vi "initialize Session Data.vi"(0 "OBJ - Session in":refnum<class "Exscalabar FPGA.lvclass">, 11 "error in":errorcluster) -> (4 "OBJ - Session out":refnum<class "Exscalabar FPGA.lvclass">, 15 "error out":errorcluster)   [LabVIEW 2014, in "Exscalabar FPGA.lvclass"]
doc: "Open an EXSCALABAR R series specific FPGA session. The system forces a wait on interrupt, so acknowledge the interrupt before moving on or the card will not respond properly. \n\nWhile the error on opening is logged, the error is further propagated so that the caller can handle the error and not just log it."
uses:
  Exscalabar FPGA.lvclass
  Exscalabar FPGA.lvclass/Exscalabar FPGA.ctl
  <vilib>/Utility/error.llb/Error Cluster From Error Code.vi
  <vilib>/rvi/errors/niLvFpgaAdjustHostInterfaceError.vi
  <vilib>/RVI Host/nirviSupport.llb/nirviErrorClusterFromErrorCode.vi
  <vilib>/rvi/interface/common/niFpgaWaitOnOcc.vi
  <vilib>/FPGAPlugInAG/PXI-7842R/niLvFpga_Open_PXI-7842R.vi
  R FPGA Ref.ctl
  <vilib>/rvi/interface/nirviMethod/nirviMethod.xnode
  FPGA Bitfiles/FPGA Server.lvbitx
  <vilib>/rvi/interface/nirviReadWriteControl/nirviReadWriteControl.xnode
  <vilib>/rvi/interface/nirviOpenFPGA/nirviOpenFPGA.xnode
  reusable/Session APIs/Session Log/System Log.lvclass
  <vilib>/rvi/errors/niLvFpgaMergeErrorWithErrorCode.vi
  <vilib>/FPGAPlugInAG/PXI-7842R/niLvFpga_ConfigureFifo_PXI-7842R.vi
  <vilib>/FPGAPlugInAG/PXI-7842R/niLvFpga_StartFifo_PXI-7842R.vi
  NiFpgaLv.dll
  <vilib>/rvi/interface/nirviMethod/StockFPGA_InlinedMethodWaitForSingleIRQ.vi
  <vilib>/FPGAPlugInAG/PXI-7842R/niLvFpga_WaitOnIrq_PXI-7842R.vi
  <vilib>/FPGAPlugInAG/PXI-7842R/niLvFpga_AcknowledgeIrq_PXI-7842R.vi
  PAS/ePAS Library.lvlib
panel:
  out "stopped":bool
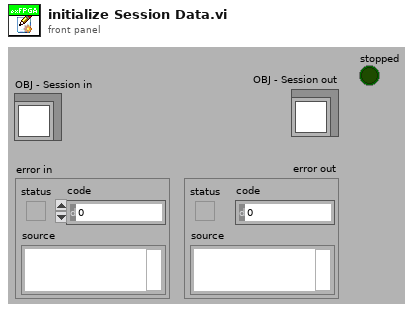
[diagram p1: front panel]
types:
  T1 = cluster{"f0":fxp<+,32,0>, "Scale":fxp<+,14,1>, "Offset":i16, "Mod":enum8{"Sine", "Square"}}
  T2 = cluster{"Ch1":bool, "Ch2":bool, "Ch3":bool, "Ch4":bool, "Ch5":bool}
  T3 = typedef "Session - Root.lvclass/Session Handle.ctl" = refnum<data-value>
  T4 = typedef "ePAS Library.lvlib/R FPGA Ref.ctl" = refnum<k20>
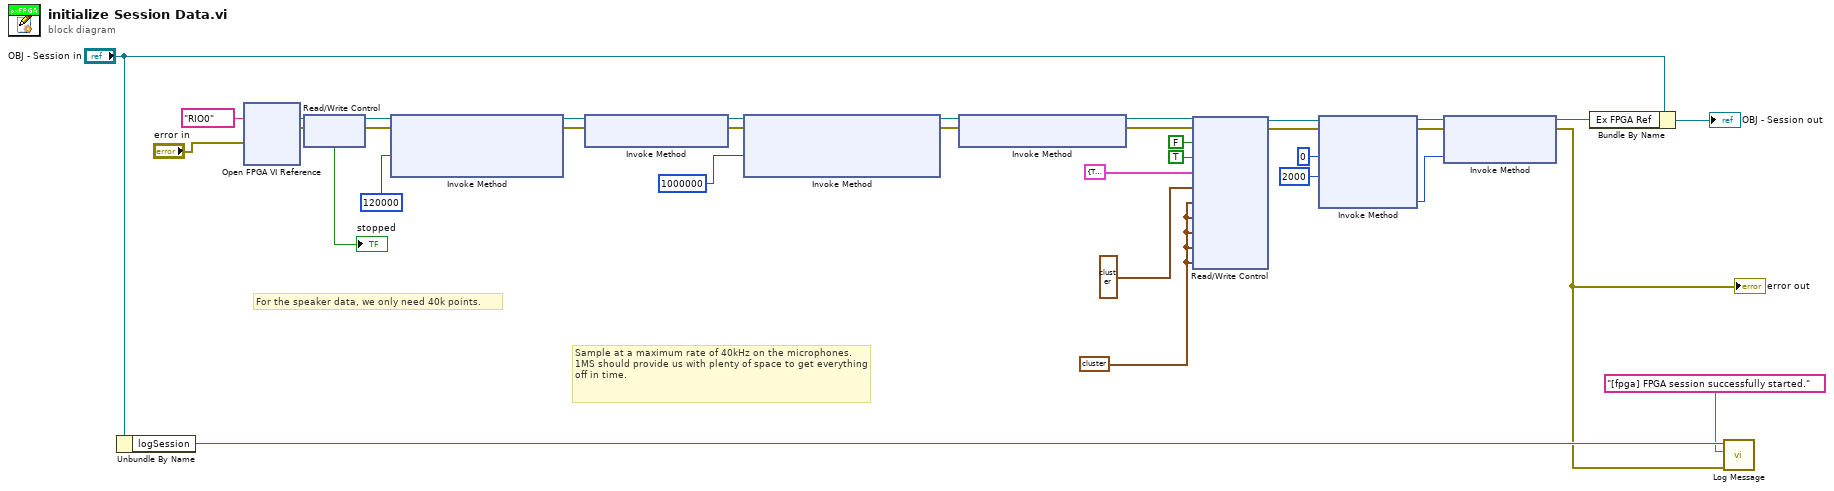
[diagram p0: block diagram]
diagram:
  w6 = T1 {"f0"=0.9999999997671694, "Scale"=1.9998779296875, "Offset"=1, "Mod"=enum."Sine"} ("Cell 5")
  # "Sample at a maximum rate of 40kHz on the microphones.  1MS should provide us with plenty of space to get everything off in time."
  # "For the speaker data, we only need 40k points."
  n1 = Unbundle By Name("OBJ - Session in") -> ("logSession"=w27:T3)
  n2 = xnode "Open FPGA VI Reference"("error in"="error in", "resource name"=tag "RIO0") -> ("FPGA VI Reference Out"=w5:T4, "error out"=w3:errorcluster)
  n3 = xnode "Read/Write Control"("FPGA VI Reference In"=w5, "error in"=w3) -> ("FPGA VI Reference Out"=w4:T4, "error out"=w1:errorcluster, "stopped"=→"stopped":bool)
  n4 = xnode "Invoke Method"("FPGA VI Reference In"=w4, "error in"=w1, "Requested Depth"=u32 120000) -> ("FPGA VI Reference Out"=w21:T4, "error out"=w20:errorcluster)  [unwired: 1 out]
  n5 = xnode "Invoke Method"("FPGA VI Reference In"=w21, "error in"=w20) -> ("FPGA VI Reference Out"=w17:T4, "error out"=w10:errorcluster)
  n6 = xnode "Invoke Method"("FPGA VI Reference In"=w17, "error in"=w10, "Requested Depth"=u32 1000000) -> ("FPGA VI Reference Out"=w18:T4, "error out"=w19:errorcluster)  [unwired: 1 out]
  n7 = xnode "Invoke Method"("FPGA VI Reference In"=w18, "error in"=w19) -> ("FPGA VI Reference Out"=w15:T4, "error out"=w14:errorcluster)
  n8 = xnode "Read/Write Control"("FPGA VI Reference In"=w15, "error in"=w14, "stop"=FALSE, "Spk Enable"=TRUE, "LaserEn"=T2 {"Ch1"=TRUE, "Ch2"=TRUE, "Ch3"=TRUE, "Ch4"=TRUE, "Ch5"=TRUE}, "Speaker"=cluster{"Voltage":fxp<+,14,1>, "Offset":i16} {"Voltage"=1.0, "Offset"=0}, "Cell 5"=w6, "Cell 4"=w6, "Cell 3"=w6, "Cell 2"=w6, "Cell 1"=w6) -> ("FPGA VI Reference Out"=w12:T4, "error out"=w11:errorcluster)
  n9 = xnode "Invoke Method"("FPGA VI Reference In"=w12, "error in"=w11, "IRQ Number(s)"=0, "Timeout (ms)"=2000) -> ("FPGA VI Reference Out"=w32:T4, "error out"=w31:errorcluster, "IRQ(s) Asserted"=w30:i32)  [unwired: 1 out]
  n10 = xnode "Invoke Method"("FPGA VI Reference In"=w32, "error in"=w31, "IRQ Number(s)"=w30) -> ("FPGA VI Reference Out"=w29:T4, "error out"=w23:errorcluster)
  "error out" <- w23
  n11 = Bundle By Name(cluster="OBJ - Session in", "Ex FPGA Ref"=w29) -> (→"OBJ - Session out":refnum<class "Exscalabar FPGA.lvclass">)
  n12 = call "Log Message.vi"("error in"=w23, "MSG In"="[fpga] FPGA session successfully started.", "session in"=w27) -> ()  [unwired: 7 in, 2 out]
